vi "LobbyPanel.vi"() -> ()   [LabVIEW 2025]
uses:
  <vilib>/Utility/miscctls.llb/LVPointTypeDef.ctl
  <vilib>/Utility/miscctls.llb/LVMapReplaceAction.ctl
  ClientGlobalVariables.vi
panel:
  out "Ready Status String":string
  in  "Ready Button":bool
  in  "mountain_density":i32(slide)=50 scale=20.0..80.0
  in  "city_density":i32(slide)=50 scale=20.0..80.0
  in  "speed":i32(slide) scale=1.0..4.0
  in  "height":i32(slide)=20 scale=20.0..40.0
  in  "width":i32(slide)=20 scale=20.0..40.0
  out "isHost?":bool
  out "Team List Display":picture
  in  "Team Buttons":T1
  # "Select your team"
  # "Options"
  # "Width:"
  # "Height:"
  # "Speed:"
  # "City Density:"
  # "Mountain Density:"
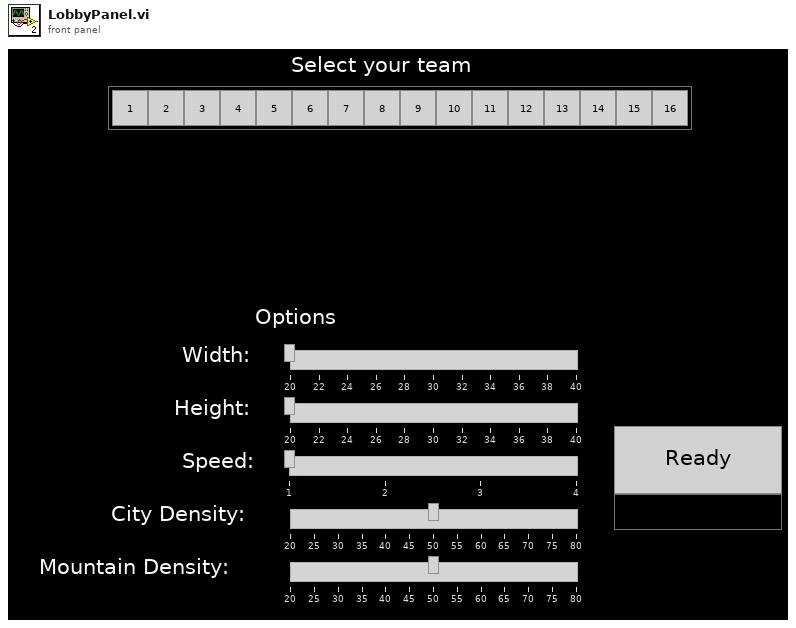
[diagram p1: front panel]
types:
  T1 = cluster{"Team Button 1":bool, "Team Button 2":bool, "Team Button 3":bool, "Team Button 4":bool, "Team Button 5":bool, "Team Button 6":bool, "Team Button 7":bool, "Team Button 8":bool, "Team Button 9":bool, "Team Button 10":bool, "Team Button 11":bool, "Team Button 12":bool, "Team Button 13":bool, "Team Button 14":bool, "Team Button 15":bool, "Team Button 16":bool}
  T2 = typedef "LVPointTypeDef.ctl" = cluster{"Horizontal":i16, "Vertical":i16}
  T3 = cluster{"ID":u32, "Name":string, "Team":u8, "Ready":bool, "Host":bool, "Alive":bool, "Color":u32, "Lands":set{cluster{"Row":u32, "Column":u32}}, "Army":u32}[]
  T4 = enum8{"Enabled", "Disabled", "Disabled and Grayed Out"}
  T5 = typedef "LVMapReplaceAction.ctl" = enum32{"Modify Entry only if found", "Add or Modify Entry", "Delete Entry"}
  T6 = cluster{"left":i16, "top":i16, "right":i16, "bottom":i16}
  T7 = cluster{"horizontal":enum16{"left", "center", "right"}, "vertical":enum16{"top", "center", "bottom"}}
  T8 = map{u8, cluster{"ID":u32, "Name":string, "Team":u8, "Ready":bool, "Host":bool, "Alive":bool, "Color":u32, "Lands":set{cluster{"Row":u32, "Column":u32}}, "Army":u32}[]}
  T9 = cluster{"Team":u8, "Team Member Array":cluster{"ID":u32, "Name":string, "Team":u8, "Ready":bool, "Host":bool, "Alive":bool, "Color":u32, "Lands":set{cluster{"Row":u32, "Column":u32}}, "Army":u32}[]}
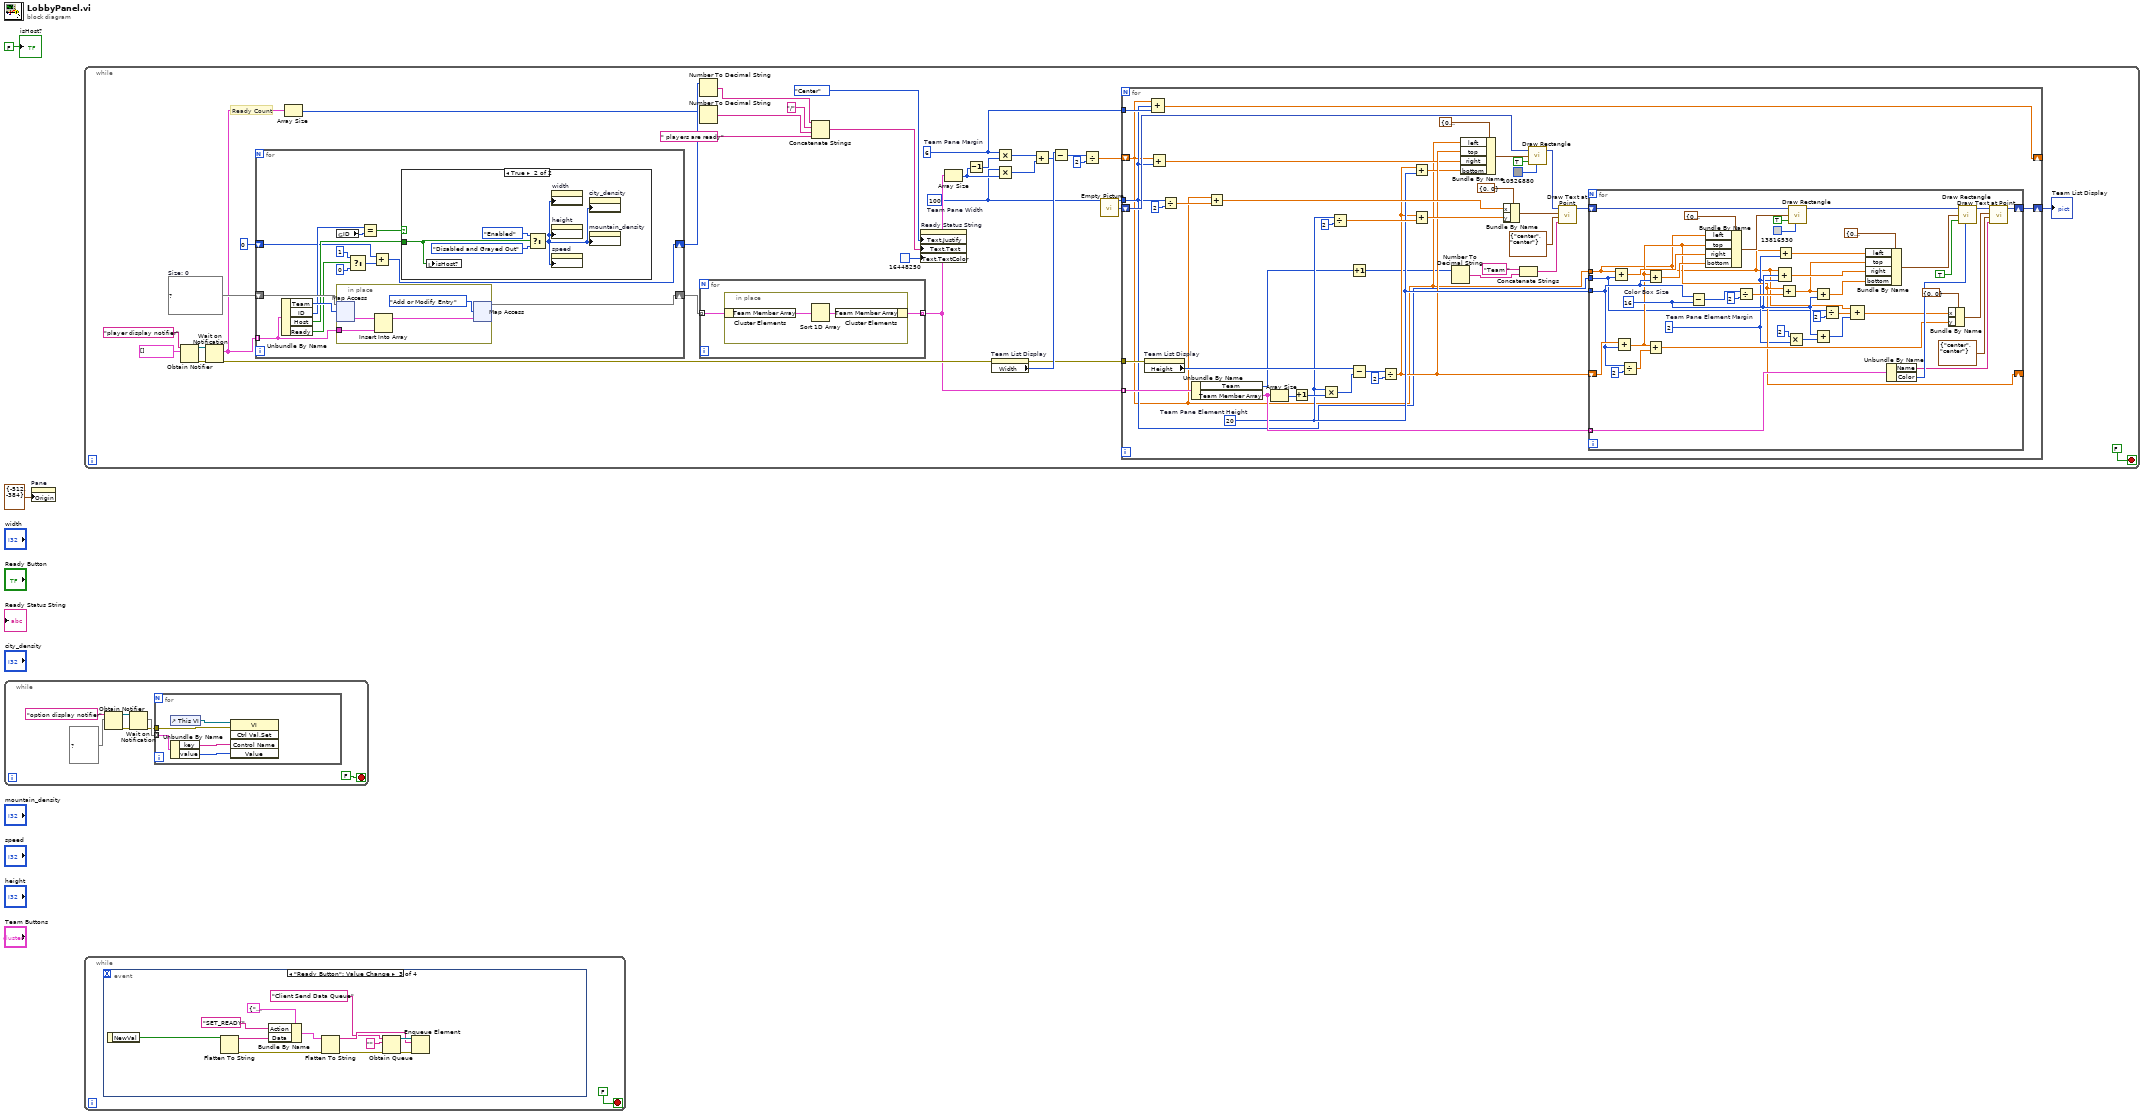
[diagram p0: block diagram]
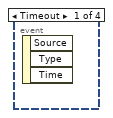
[diagram p2: hidden frame]
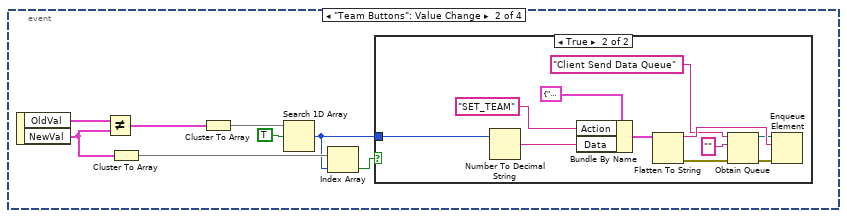
[diagram p3: hidden frame]
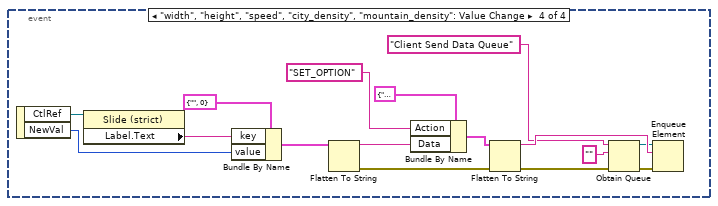
[diagram p5: hidden frame]
diagram:
  n1 = while {
    stop <- FALSE stop-if-true
    n2 = Obtain Notifier(name (unnamed)="option display notifier", notification data type=map{string, i32} {} ("Options")) -> (notifier out=w4:refnum<notifier>, error out=w3:errorcluster)  [unwired: 2 in, 1 out]
    n3 = Wait on Notification(notifier=w4, error in (no error)=w3) -> (notification=w9:map{string, i32}, error out=w8:errorcluster)  [unwired: 2 in, 2 out]
    n4 = for {
      tunnel: w9 -> [w14] mode=indexing
      tunnel: w8 -> [w10]
      n5 = control-ref of="This VI"() -> (w11:refnum<vi>)
      n6 = Unbundle By Name(w14) -> ("key"=w13:string, "value"=w12:i32)
      n7 = invoke on="Invoke Node" class="VI" method="Ctrl Val.Set"(reference=w11, error in=w10, "Control Name"=w13, "Value"=w12) -> ()  [unwired: 1 in, 5 out]
    }
  }
  n8 = property on="Pane" class="Pane"("Origin"=T2 {"Horizontal"=-512, "Vertical"=-384}) -> ()  [unwired: 2 in, 2 out]
  n9 = while {
    stop <- FALSE stop-if-true
    w22 = T8 {}  # Size: 0
    w34 = 6  # Team Pane Margin
    w35 = 100  # Team Pane Width
    # "Ready Count"
    n10 = Obtain Notifier(name (unnamed)="player display notifier", notification data type=T3 [] ("PlayerInfoArray")) -> (notifier out=w27:refnum<notifier>, error out=w28:errorcluster)  [unwired: 2 in, 1 out]
    n11 = Wait on Notification(notifier=w27, error in (no error)=w28) -> (notification=w15:T3, error out=w48:errorcluster)  [unwired: 2 in, 2 out]
    n12 = for {
      tunnel: w15 -> [w64] mode=indexing
      shift-right: [w63] -> w44
      shift-left: w22 -> [w66]
      shift-right: [w54] -> w24
      shift-left: 0 -> [w53]
      n13 = Unbundle By Name(w64) -> ("Team"=w65:u8, "ID"=w62:u32, "Host"=w59:bool, "Ready"=w58:bool)
      n14 = global read "ClientGlobalVariables.vi" "ID"() -> (w61:u32)
      n15 = in-place {
        in-place-border: w64 -> [w73]
        n16 = in-place-map #1(w66, w65) -> (w74:T3)  [unwired: 1 in, 1 out]
        n17 = Insert Into Array(array=w74, new element=w73) -> (w72:T3)  [unwired: 1 in]
        n18 = in-place-map #1(w72, LVMapReplaceAction."Add or Modify Entry" ("action")) -> (w63:T8)  [unwired: 2 out]
      }
      n19 = Select(t=1, s=w58, f=0) -> (s? t:f=w55:i32)
      n20 = Equal?(x=w62, y=w61) -> (x = y?=w60:bool)
      n21 = Add(x=w53, y=w55) -> (x+y=w54:i32)
      n22 = case shown="True" w60 {
        tunnel: w59 -> [_ w70]
        frame False {
        }
        frame True {
          n23 = local write "isHost?"(w70) -> ()
          n24 = Select(t=T4."Enabled" ("Disabled"), s=w70, f=T4."Disabled and Grayed Out" ("Disabled")) -> (s? t:f=w67:T4)
          n25 = property on="width" class="Slide (strict)"("DisabledEnum"=w67) -> ()  [unwired: 2 in, 2 out]
          n26 = property on="height" class="Slide (strict)"("DisabledEnum"=w67) -> ()  [unwired: 2 in, 2 out]
          n27 = property on="speed" class="Slide (strict)"("DisabledEnum"=w67) -> ()  [unwired: 2 in, 2 out]
          n28 = property on="city_density" class="Slide (strict)"("DisabledEnum"=w67) -> ()  [unwired: 2 in, 2 out]
          n29 = property on="mountain_density" class="Slide (strict)"("DisabledEnum"=w67) -> ()  [unwired: 2 in, 2 out]
        }
      }
    }
    n30 = Array Size(array=w15) -> (size(s)=w21:i32)
    n31 = Number To Decimal String(number=w24) -> (decimal integer string=w23:string)  [unwired: 1 in]
    n32 = Number To Decimal String(number=w21) -> (decimal integer string=w20:string)  [unwired: 1 in]
    n33 = for {
      tunnel: w44 -> [w50] mode=indexing
      tunnel: [w49] -> w36 mode=indexing
      n34 = in-place {
        n35 = in-place-cluster #2(w50) -> ("Team Member Array"=w52:T3)
        n36 = Sort 1D Array(array=w52) -> (sorted array=w51:T3)
        n37 = in-place-cluster #2("Team Member Array"=w51) -> (w49:T9)
      }
    }
    n38 = Concatenate Strings(w23, "/" ("string"), w20, " players are ready" ("string")) -> (w17:string)
    n39 = property on="Ready Status String" class="Str"("Text.Justify"=enum16{"Left", "Center", "Right"}."Center" ("Text.Justification"), "Text.Text"=w17, "Text.TextColor"=u32 16448250 ("Text.Text Colors:Text Color")) -> ()  [unwired: 2 in, 2 out]
    n40 = Array Size(array=w36) -> (size(s)=w45:i32)
    n41 = Decrement(x=w45) -> (x-1=w46:i32)
    n42 = property on="Team List Display" class="Pict"(error in=w48) -> (error out=w38:errorcluster, "Width"=w42:u32)  [unwired: 1 in, 1 out]
    n43 = Multiply(x=w34, y=w46) -> (x*y=w41:i32)
    n44 = Multiply(x=w35, y=w45) -> (x*y=w31:i32)
    n45 = Add(x=w41, y=w31) -> (x+y=w32:i32)
    n46 = Subtract(x=w42, y=w32) -> (x-y=w40:u32)
    n47 = Divide(x=w40, y=u32 2) -> (x/y=w39:dbl)
    n48 = call "Empty Picture"() -> ("empty picture"=w37:picture)
    n49 = for {
      tunnel: w38 -> [w113]
      shift-right: [w112] -> _
      shift-left: w39 -> [w77]
      tunnel: w35 -> [w79]
      shift-right: [w89] -> w33
      shift-left: w37 -> [w84]
      tunnel: w36 -> [w111] mode=indexing
      tunnel: w34 -> [w100]
      w82 = 20  # Team Pane Element Height
      n50 = property on="Team List Display" class="Pict"(error in=w113) -> ("Height"=w109:u32)  [unwired: 1 in, 2 out]
      n51 = Add(x=w77, y=w79) -> (x+y=w78:dbl)
      n52 = Compound Arithmetic op=ADD(w77, w79, w100) -> (w112:dbl)
      n53 = Divide(x=w79, y=2) -> (x/y=w97:dbl)
      n54 = Unbundle By Name(w111) -> ("Team"=w76:u8, "Team Member Array"=w93:T3)
      n55 = Add(x=w77, y=w97) -> (x+y=w91:dbl)
      n56 = Array Size(array=w93) -> (size(s)=w110:i32)
      n57 = Increment(x=w110) -> (x+1=w105:i32)
      n58 = Multiply(x=w82, y=w105) -> (x*y=w108:i32)
      n59 = Divide(x=w82, y=u32 2) -> (x/y=w95:dbl)
      n60 = Increment(x=w76) -> (x+1=w75:u8)
      n61 = Subtract(x=w109, y=w108) -> (x-y=w106:u32)
      n62 = Divide(x=w106, y=u32 2) -> (x/y=w81:dbl)
      n63 = Add(x=w81, y=w82) -> (x+y=w80:dbl)
      n64 = Add(x=w81, y=w95) -> (x+y=w90:dbl)
      n65 = Number To Decimal String(number=w75) -> (decimal integer string=w102:string)  [unwired: 1 in]
      n66 = Bundle By Name(cluster=T6 {"left"=0, "top"=0, "right"=0, "bottom"=0} ("rect"), "left"=w77, "top"=w81, "right"=w78, "bottom"=w80) -> (w86:T6)
      n67 = Bundle By Name(cluster=cluster{"x":i16, "y":i16} {"x"=0, "y"=0} ("origin"), "x"=w91, "y"=w90) -> (w94:cluster{"x":i16, "y":i16})
      n68 = Concatenate Strings("Team " ("string"), w102) -> (w101:string)
      n69 = call <vilib>:"Draw Rectangle.vi"("picture"=w84, "rect"=w86, "fill?(F)"=TRUE, "color(black)"=u32 10526880) -> ("new picture"=w83:picture)  [unwired: 5 in]
      n70 = call <vilib>:"Draw Text at Point.vi"("text"=w101, "alignment(left, top)"=T7 {"horizontal"=enum."center", "vertical"=enum."center"}, "origin"=w94, "picture"=w83) -> ("new picture"=w92:picture)  [unwired: 6 in, 1 out]
      n71 = for {
        tunnel: w93 -> [w155] mode=indexing
        shift-right: [w143] -> w89
        shift-left: w92 -> [w130]
        tunnel: w77 -> [w118]
        tunnel: w82 -> [w124]
        shift-right: [w122] -> _
        shift-left: w81 -> [w125]
        tunnel: w79 -> [w117]
        w140 = u32 16  # Color Box Size
        w119 = u32 2  # Team Pane Element Margin
        n72 = Add(x=w118, y=w117) -> (x+y=w126:dbl)
        n73 = Add(x=w125, y=w124) -> (x+y=w122:dbl)
        n74 = Divide(x=w124, y=2) -> (x/y=w133:dbl)
        n75 = Add(x=w122, y=w124) -> (x+y=w123:dbl)
        n76 = Add(x=w122, y=w133) -> (x+y=w132:dbl)
        n77 = Subtract(x=w124, y=w140) -> (x-y=w149:u32)
        n78 = Bundle By Name(cluster=T6 {"left"=0, "top"=0, "right"=0, "bottom"=0} ("rect"), "left"=w118, "top"=w122, "right"=w126, "bottom"=w123) -> (w127:T6)
        n79 = Divide(x=w149, y=2) -> (x/y=w148:dbl)
        n80 = Add(x=w118, y=w119) -> (x+y=w120:dbl)
        n81 = Compound Arithmetic op=unknown(w118, w140, w119) -> (w151:dbl)
        n82 = Add(x=w122, y=w148) -> (x+y=w147:dbl)
        n83 = Multiply(x=u32 2, y=w119) -> (x*y=w138:u32)
        n84 = call <vilib>:"Draw Rectangle.vi"("picture"=w130, "rect"=w127, "fill?(F)"=TRUE, "color(black)"=u32 13816530) -> ("new picture"=w131:picture)  [unwired: 5 in]
        n85 = Add(x=w147, y=w140) -> (x+y=w146:dbl)
        n86 = Add(x=w140, y=w138) -> (x+y=w114:u32)
        n87 = Divide(x=w117, y=2) -> (x/y=w115:dbl)
        n88 = Compound Arithmetic op=unknown(w118, w115, w114) -> (w135:dbl)
        n89 = Bundle By Name(cluster=T6 {"left"=0, "top"=0, "right"=0, "bottom"=0} ("rect"), "left"=w120, "top"=w147, "right"=w151, "bottom"=w146) -> (w145:T6)
        n90 = Unbundle By Name(w155) -> ("Name"=w141:string, "Color"=w154:u32)
        n91 = Bundle By Name(cluster=cluster{"x":i16, "y":i16} {"x"=0, "y"=0} ("origin"), "x"=w135, "y"=w132) -> (w136:cluster{"x":i16, "y":i16})
        n92 = call <vilib>:"Draw Rectangle.vi"("picture"=w131, "rect"=w145, "fill?(F)"=TRUE, "color(black)"=w154) -> ("new picture"=w144:picture)  [unwired: 5 in]
        n93 = call <vilib>:"Draw Text at Point.vi"("text"=w141, "alignment(left, top)"=T7 {"horizontal"=enum."center", "vertical"=enum."center"}, "origin"=w136, "picture"=w144) -> ("new picture"=w143:picture)  [unwired: 6 in, 1 out]
      }
    }
    "Team List Display" <- w33
  }
  n94 = while {
    stop <- FALSE stop-if-true
    n95 = event shown="[2] \"Ready Button\": Value Change" {
      selector: _ -> [_ _ _ _]
      dyn-events: _ -> [_ _ _ _]
      timeout: _ -> [_ _ _ _]
      event Timeout {
        n96 = event-data() -> ()  [unwired: 1 in, 3 out]
      }
      event "Team Buttons": Value Change {
        n97 = event-data() -> ("OldVal"=w164:T1, "NewVal"=w160:T1)  [unwired: 1 in]
        n98 = Not Equal?(x=w164, y=w160) -> (x != y?=w163:T1)
        n99 = Cluster To Array(cluster=w160) -> (array=w159:bool[])
        n100 = Cluster To Array(cluster=w163) -> (array=w162:bool[])
        n101 = Search 1D Array(1D array=w162, element=TRUE) -> (index of element=w157:i32)  [unwired: 1 in]
        n102 = Index Array(array=w159, index=w157) -> (element=w158:bool)
        n103 = case shown="True" w158 {
          tunnel: w157 -> [_ w172]
          frame False {
          }
          frame True {
            n104 = Number To Decimal String(number=w172) -> (decimal integer string=w171:string)  [unwired: 1 in]
            n105 = Bundle By Name(cluster=cluster{"Action":string, "Data":string} {"Action"="", "Data"=""} ("CommandCluster"), "Action"="SET_TEAM", "Data"=w171) -> (w174:cluster{"Action":string, "Data":string})
            n106 = Flatten To String(anything=w174) -> (data string=w173:string, error out=w167:errorcluster)  [unwired: 3 in, 1 out]
            n107 = Obtain Queue(name (unnamed)="Client Send Data Queue", element data type="", error in (no error)=w167) -> (queue out=w165:refnum<queue>, error out=w166:errorcluster)  [unwired: 2 in, 1 out]
            n108 = Enqueue Element(queue=w165, element=w173, error in (no error)=w166) -> ()  [unwired: 1 in, 3 out]
          }
        }
      }
      event "Ready Button": Value Change {
        n109 = event-data() -> ("NewVal"=w178:bool)  [unwired: 1 in]
        n110 = Flatten To String(anything=w178) -> (data string=w176:string, error out=w177:errorcluster)  [unwired: 3 in, 1 out]
        n111 = Bundle By Name(cluster=cluster{"Action":string, "Data":string} {"Action"="", "Data"=""} ("CommandCluster"), "Action"="SET_READY", "Data"=w176) -> (w183:cluster{"Action":string, "Data":string})
        n112 = Flatten To String(anything=w183, error in (no error)=w177) -> (data string=w184:string, error out=w185:errorcluster)  [unwired: 2 in, 1 out]
        n113 = Obtain Queue(name (unnamed)="Client Send Data Queue", element data type="", error in (no error)=w185) -> (queue out=w187:refnum<queue>, error out=w186:errorcluster)  [unwired: 2 in, 1 out]
        n114 = Enqueue Element(queue=w187, element=w184, error in (no error)=w186) -> ()  [unwired: 1 in, 3 out]
      }
      event "width", "height", "speed", "city_density", "mountain_density": Value Change {
        n115 = event-data() -> ("CtlRef"=w203:refnum<vi>, "NewVal"=w196:i32)  [unwired: 1 in]
        n116 = property class="Slide (strict)"(reference=w203) -> ("Label.Text"=w197:string)  [unwired: 1 in, 2 out]
        n117 = Bundle By Name(cluster=cluster{"key":string, "value":i32} {"key"="", "value"=0}, "key"=w197, "value"=w196) -> (w194:cluster{"key":string, "value":i32})
        n118 = Flatten To String(anything=w194) -> (data string=w195:string, error out=w193:errorcluster)  [unwired: 3 in, 1 out]
        n119 = Bundle By Name(cluster=cluster{"Action":string, "Data":string} {"Action"="", "Data"=""} ("CommandCluster"), "Action"="SET_OPTION", "Data"=w195) -> (w201:cluster{"Action":string, "Data":string})
        n120 = Flatten To String(anything=w201, error in (no error)=w193) -> (data string=w200:string, error out=w190:errorcluster)  [unwired: 2 in, 1 out]
        n121 = Obtain Queue(name (unnamed)="Client Send Data Queue", element data type="", error in (no error)=w190) -> (queue out=w192:refnum<queue>, error out=w191:errorcluster)  [unwired: 2 in, 1 out]
        n122 = Enqueue Element(queue=w192, element=w200, error in (no error)=w191) -> ()  [unwired: 1 in, 3 out]
      }
    }
  }
  "isHost?" <- FALSE ("isHost?")
